vi "Jaguar Sync Testbench.vi"() -> ()   [LabVIEW 2013]
doc: "This VI imlements the framework and scheduler for your robotics program. It should not be necessary to modify the framework. You are expected to add your code to the VIs called from Robot Main, the ones located in the Team Code within the project."
uses:
  <vilib>/Rock Robotics/WPI/CAN/Jaguar/SubVIs/WPI_CANJaguar_ControlMode.ctl
  <vilib>/Rock Robotics/WPI/SafetyOutput/WPI_SafetyOutputConfigMenu.ctl
panel:
  in  "Encoder Codes Per Rev":u16=256
  in  "Target":dbl=2.0
  in  "PID gains":T1={"proportional gain (Kp)"=50.0, "integral gain (Ki)"=0.1, "derivative gain (Kd)"=40.0}
  in  "Start":bool
  in  "Finish":bool
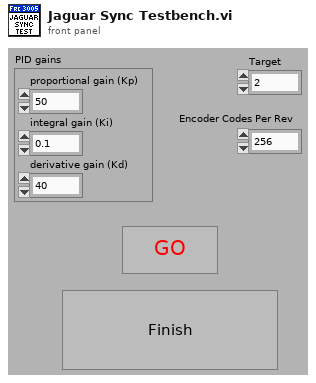
[diagram p1: front panel]
types:
  T1 = cluster{"proportional gain (Kp)":dbl, "integral gain (Ki)":dbl, "derivative gain (Kd)":dbl}
  T2 = typedef "WPI_SafetyOutputConfigMenu.ctl" = enum16{"Enable", "Disable"}
  T3 = typedef "WPI_CANJaguar_ControlMode.ctl" = enum8{"Percent VBus", "Current", "Speed", "Position", "Voltage"}
  T4 = typedef "WPI_RobotDriveDevRef.ctl" = cluster{"DevStatus":errorcluster, "Motors[]":T5[], "Square Inputs":bool, "Max Output":dbl, "Isochronous":bool}
  T5 = typedef "WPI_MotorControlDeviceRef.ctl" = cluster{"DeviceStatus":errorcluster, "Type":enum16{"PWM", "CAN"}, "PWM":cluster{"Digital Module":T6, "PWM Channel":T7, "DeadBand":T8}, "CAN":cluster{"Device Number":u8, "Control Mode":T3, "Semaphore":T9, "Max Vout":dbl}, "Invert":bool, "TransformRef":T10, "InvTransformRef":T10}
  T6 = typedef "FPGA_TypedefDigitalModule.ctl" = enum16{"Digital Module 1", "Digital Module 2"}
  T7 = typedef "FPGA_DIOPWMChannel.ctl" = enum8{"PWM 1", "PWM 2", "PWM 3", "PWM 4", "PWM 5", "PWM 6", "PWM 7", "PWM 8", "PWM 9", "PWM 10", "Invalid"}
  T8 = typedef "WPI_PWMDeadband.ctl" = cluster{"Name":string, "maxPositivePwm":i32, "minPositivePwm":i32, "centerPwm":i32, "maxNegativePwm":i32, "minNegativePwm":i32, "angularRange":u16}
  T9 = typedef "Semaphore RefNum" = refnum<k1>
  T10 = typedef "WPI_PWMTransform_ConPane.ctl" = refnum<vi>
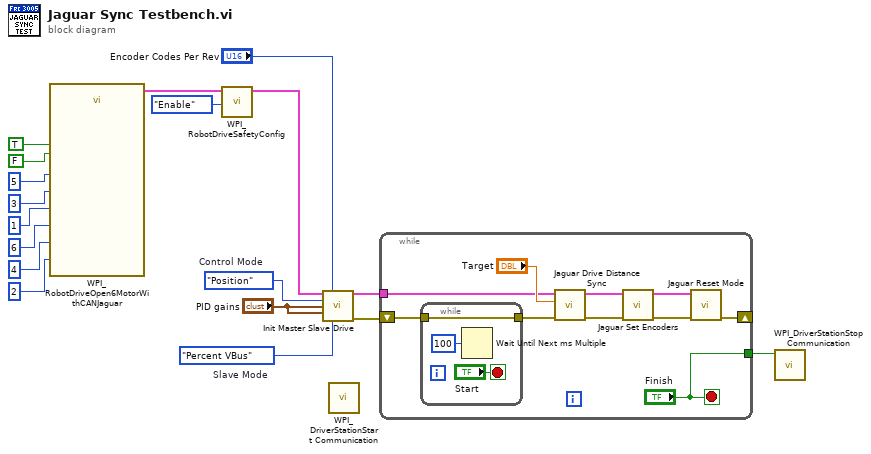
[diagram p0: block diagram]
diagram:
  w18 = WPI_CANJaguar_ControlMode."Percent VBus"  # Slave Mode
  w17 = WPI_CANJaguar_ControlMode."Position"  # Control Mode
  n1 = call <vilib>:"WPI_RobotDriveOpen6MotorWithCANJaguar.vi"("Rear Left Motor"=u8 1, "Rear Right Motor"=u8 2, "Front Right Motor"=u8 6, "Front Left Motor"=u8 5, "Mid Left Motor"=u8 3, "Mid Right Motor"=u8 4, "Left Motors Inverted"=TRUE, "Right Motors Inverted"=FALSE) -> ("RobotDriveDevRef"=w2:T4)  [unwired: 10 in, 1 out]
  n2 = call <vilib>:"WPI_RobotDriveSafetyConfig.vi"("mode"=WPI_SafetyOutputConfigMenu."Enable", "RobotDriveDevRef"=w2) -> ("RobotDriveDevRef"=w1:T4)  [unwired: 8 in, 1 out]
  n3 = call "Init Master Slave Drive.vi"("RobotDriveDevRef"=w1, "Encoder Codes Per Rev"="Encoder Codes Per Rev", "Control Mode"=w17, "Left PID gains"="PID gains", "Right PID gains"="PID gains", "Slave Mode"=w18) -> ("RobotDriveDevRef Out"=w15:T4, "error out"=w14:errorcluster)  [unwired: 8 in]
  n4 = call <vilib>:"WPI_DriverStationStart Communication.vi"() -> ()  [unwired: 12 in]
  n5 = while {
    tunnel: w15 -> [w23]
    shift-right: [w22] -> _
    shift-left: w14 -> [w21]
    tunnel: ["Finish"] -> w12
    stop <- "Finish" stop-if-true
    n6 = while {
      tunnel: w21 -> [w29]
      tunnel: [w29] -> w20
      stop <- "Start" stop-if-true
      n7 = Wait Until Next ms Multiple(millisecond multiple=u32 100) -> ()  [unwired: 1 out]
    }
    n8 = call "Jaguar Drive Distance Sync.vi"("error in (no error)"=w20, "Rotations"="Target", "RobotDriveDevRef"=w23) -> ("error out"=w27:errorcluster, "RobotDriveDevRef Out"=w26:T4)  [unwired: 7 in]
    n9 = call "Jaguar Set Encoders.vi"("error in"=w27, "RobotDriveDevRef"=w26) -> ("error out"=w24:errorcluster, "RobotDriveDevRef Out"=w25:T4)  [unwired: 8 in]
    n10 = call "Jaguar Reset Mode.vi"("error in"=w24, "RobotDriveDevRef"=w25) -> ("error out"=w22:errorcluster)  [unwired: 8 in, 1 out]
  }
  n11 = call <vilib>:"WPI_DriverStationStop Communication.vi"("StopCommunication"=w12) -> ()  [unwired: 10 in, 1 out]
